vi "Process Incoming Messages.vi"(0 "J1939 Cluster":T11, 1 "Addresses":u8[](array[numeric]), 5 "CAN frame":T9 {"payload" format="%x"; "timestamp" format="%<%.7X\n%x>T"; "type" items=["CAN Data"=0, "CAN Remote"=1, "CAN Bus Error"=2, "CAN 2.0 Data"=8, "CAN FD Data"=16, "CAN FD+BRS Data"=24, "J1939 Data"=192, "Delay"=224, "Log Trigger"=225, "Start Trigger"=226]; "identifier" format="%x"}, 7 "ref in":T3, 9 "Simulated Addresses LUT":variant, 11 "error in":errorcluster, 12 "Scale Ref":T2, 13 "Data Ref":T1) -> (4 "J1939 Cluster Out":T11, 15 "error out":errorcluster)   [LabVIEW 2015, in "J1939 Addon Engine.lvlib"]
uses:
  Engine/J1939 Addon Engine.lvlib
  Types/Setup Information Cluster.ctl
  <vilib>/xnet/xnet.llb/XNET Frame CAN.ctl
  <vilib>/xnet/xnet.llb/XNET Frame Type CAN.ctl
  J1939 Utilities/Types/CAN Outgoing Message Cluster.ctl
  Types/TP List References.ctl
  Types/BAM Buffer Connections List_Ref.ctl
  Types/TP Buffer Connection Cluster.ctl
  Types/Connection Mode Generation Connection Ref.ctl
  Types/Connection Mode Generation Connection Cluster.ctl
  Types/BAM Generation Connections List_Ref.ctl
  Types/BAM Generation Connection Cluster.ctl
  Types/Address Table Reference.ctl
  Types/RQST Lookup Table Reference.ctl
  Engine/Types/Conversion Lookup Table Reference.ctl
  Engine/Types/Data Lookup Table Reference.ctl
  Engine/Types/Datatable Lookup DVR.ctl
  J1939 Utilities/Parse Message Type.vi
  SubVIs/RQST Lookup Table Act.vi
  J1939 Utilities/Common Conversions.vi
  J1939 Utilities/SubVIs/Convert CAN Arb ID to J1939 ID.vi
  J1939 Utilities/SubVIs/Convert J1939 ID to CAN Arb ID.vi
  J1939 Utilities/SubVIs/Convert CAN Data (U32) to U8.vi
  Engine/SubVIs/Get Simulated Previously Active DTCs.vi
  Engine/SubVIs/Get Simulated Active DTCs.vi
  J1939 Utilities/Common Messages.vi
  J1939 Utilities/SubVIs/Acknowledgement.vi
  Engine/SubVIs/Send Reset Previously Active DTC to Main.vi
  Engine/SubVIs/Send Reset Active DTC to Main.vi
  Engine/SubVIs/Convert Signals to Frame by ID.vi
  J1939 Multi Packet Frames/BAM Buffer.vi
  SubVIs/Buffer Connections List_Actions.vi
  SubVIs/TP Buffer Search for Connection (No PGN).vi
  SubVIs/TP Buffer Add New Data Packet to Connection.vi
  SubVIs/TP Buffer Convert Connection Info to CAN Frame.vi
  SubVIs/TP Buffer Create New TP Connection.vi
  J1939 Multi Packet Frames/Connnection Mode Buffer.vi
  J1939 Utilities/SubVIs/TP.CM EndofMsgACK.vi
  J1939 Utilities/SubVIs/TP.CM CTS.vi
  J1939 Utilities/SubVIs/TP.Conn Abort.vi
  J1939 Multi Packet Frames/Connection Mode Generation.vi
  SubVIs/Connection Mode Generation Connections List_Actions.vi
  SubVIs/Connection Mode Generation Search for Connection (Remote Message).vi
  SubVIs/TP Buffer Search for Connection.vi
  SubVIs/Connection Mode Generation CTS Received.vi
  Engine/SubVIs/Network Address Lookup Table.vi
  Engine/SubVIs/Convert Data to DTC Frame.vi
  Engine/SubVIs/Conversion Lookup Table Get Conversion Parameter.vi
  Engine/SubVIs/Data Lookup Table Get Signals (Range).vi
  J1939 Utilities/SubVIs/Convert PGN + SA to J1939 ID.vi
  SubVIs/Address Lookup Table.vi
  SubVIs/BAM Buffer Connections List.vi
  SubVIs/Connection Mode Generation Connections List.vi
  <vilib>/xnet/xnet.llb/XNET Convert.vi
  <vilib>/xnet/xnet.llb/XNET Convert (Signal to Frame Raw).vi
  Engine/SubVIs/Data Lookup Table.vi
  Engine/SubVIs/Conversion Lookup Table.vi
  SubVIs/RQST Lookup Table.vi
  J1939 Utilities/J1939 Utilities.lvlib
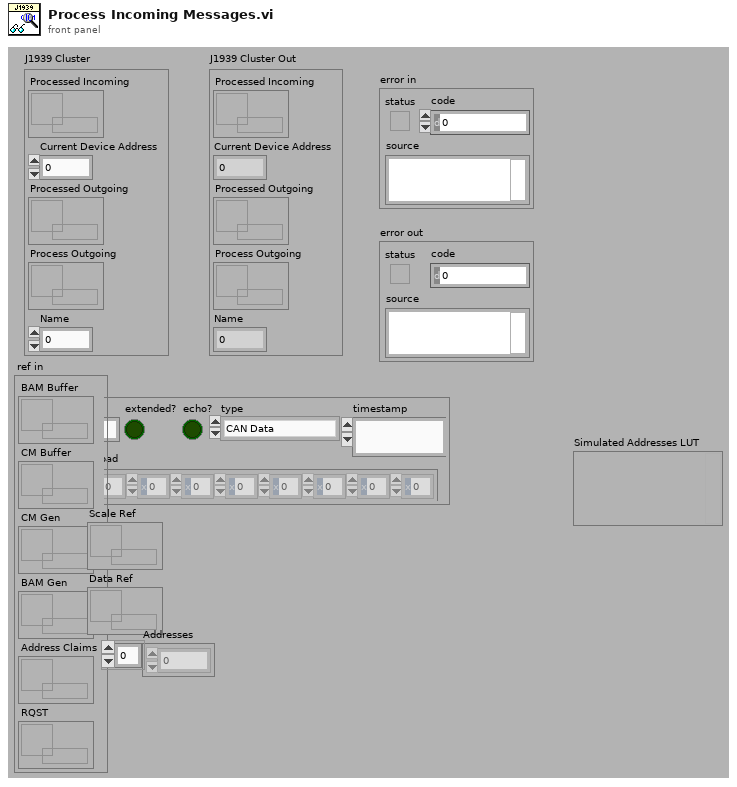
[diagram p1: front panel]
types:
  T1 = typedef "J1939 Addon Engine.lvlib/Data Lookup Table Reference.ctl" = refnum<data-value>
  T2 = typedef "J1939 Addon Engine.lvlib/Conversion Lookup Table Reference.ctl" = refnum<data-value>
  T3 = typedef "J1939 Addon Engine.lvlib/TP List References.ctl" = cluster{"BAM Buffer":T4, "CM Buffer":T4, "CM Gen":T5, "BAM Gen":T6, "Address Claims":T7, "RQST":T8}
  T4 = typedef "J1939 Addon Engine.lvlib/BAM Buffer Connections List_Ref.ctl" = refnum<data-value>
  T5 = typedef "J1939 Addon Engine.lvlib/Connection Mode Generation Connection Ref.ctl" = refnum<data-value>
  T6 = typedef "J1939 Addon Engine.lvlib/BAM Generation Connections List_Ref.ctl" = refnum<data-value>
  T7 = typedef "J1939 Addon Engine.lvlib/Address Table Reference.ctl" = refnum<data-value>
  T8 = typedef "J1939 Addon Engine.lvlib/RQST Lookup Table Reference.ctl" = refnum<data-value>
  T9 = typedef "XNET Frame CAN.ctl" = cluster{"timestamp":timestamp, "payload":u8[], "identifier":u32, "type":T10, "extended?":bool, "echo?":bool}
  T10 = typedef "XNET Frame Type CAN.ctl" = u8
  T11 = typedef "J1939 Addon Engine.lvlib/Setup Information Cluster.ctl" = cluster{"Processed Incoming":refnum<queue>, "Current Device Address":u8, "Processed Outgoing":refnum<queue>, "Process Outgoing":refnum<queue>, "Name":u64}
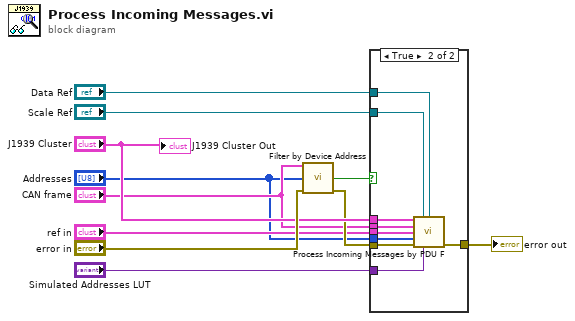
[diagram p0: block diagram]
diagram:
  n1 = call "Filter by Device Address.vi"("CAN Frame"="CAN frame", "Addresses"="Addresses", "error in"="error in") -> ("Pass Through"=w9:bool, "error out"=w8:errorcluster)  [unwired: 11 out]
  n2 = case shown="True" w9 {
    tunnel: [w12 w21] -> w7
    tunnel: w8 -> [w12 w20]
    tunnel: "CAN frame" -> [_ w17]
    tunnel: "J1939 Cluster" -> [_ w18]
    tunnel: "ref in" -> [_ w19]
    tunnel: "Scale Ref" -> [_ w16]
    tunnel: "Data Ref" -> [_ w15]
    tunnel: "Addresses" -> [_ w14]
    tunnel: "Simulated Addresses LUT" -> [_ w13]
    frame False {
    }
    frame True {
      n3 = call "Process Incoming Messages by PDU F.vi"("J1939 Cluster"=w18, "Scale Ref"=w16, "Data Ref"=w15, "CAN frame"=w17, "ref in"=w19, "Addresses"=w14, "error in"=w20, "Simulated Addresses LUT"=w13) -> ("error out"=w21:errorcluster)  [unwired: 7 out]
    }
  }
  "error out" <- w7
  "J1939 Cluster Out" <- "J1939 Cluster"
